vi "Header Title.vi"(8 "Error In":errorcluster, 10 "Header Title":string, 11 "String in":string) -> (0 "Error Out":errorcluster, 3 "String out":string)   [LabVIEW 2018]
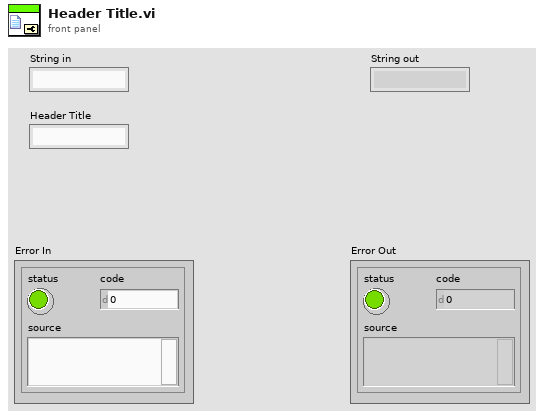
[diagram p1: front panel]
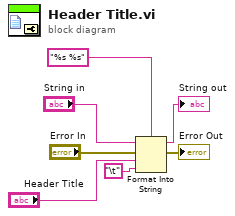
[diagram p0: block diagram]
diagram:
  n1 = Format Into String(format string="%s %s", initial string="String in", error in="Error In", "Header Title", "\t") -> (resulting string=→"String out":string, error out=→"Error Out":errorcluster)
